vi "CollectPoint.vi"(8 "error in (no error)":errorcluster, 11 "Snake in":refnum<class "SnakeGame.lvclass">) -> (0 "error out":errorcluster, 3 "Snake out":refnum<class "SnakeGame.lvclass">)   [LabVIEW 2019, in "RT_Game.lvlib" / "SnakeGame.lvclass"]
uses:
  SnakeGame.lvclass
  SnakeGame.lvclass/SnakeGame.ctl
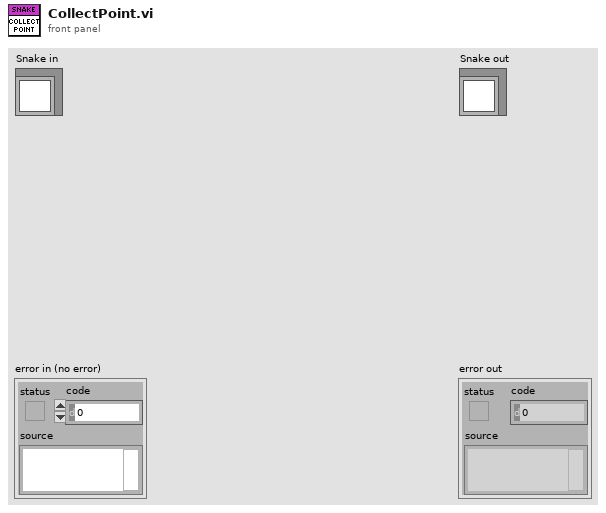
[diagram p1: front panel]
types:
  T1 = typedef "RT_Game.lvlib/Game.lvclass/Coordinate.ctl" = cluster{"x":dbl, "y":dbl}
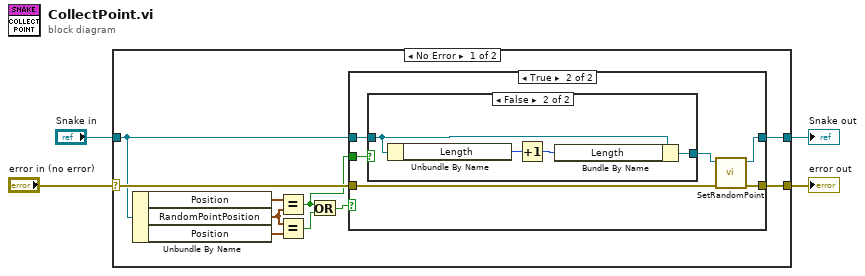
[diagram p0: block diagram]
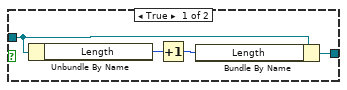
[diagram p3: hidden frame]
diagram:
  n1 = case shown="No Error" "error in (no error)" {
    selector: "error in (no error)" -> [w14 w32]
    tunnel: [w12 w32] -> w3
    tunnel: [w11 w31] -> w1
    tunnel: "Snake in" -> [w10 w31]
    frame No Error {
      n2 = Unbundle By Name(w10) -> ("Position"=w13:T1, "RandomPointPosition"=w9:T1, "Position"=w8:T1)
      n3 = Equal?(x=w13, y=w9) -> (x = y?=w5:bool)
      n4 = Equal?(x=w9, y=w8) -> (x = y?=w6:bool)
      n5 = Or(x=w5, y=w6) -> (x .or. y?=w7:bool)
      n6 = case shown="True" w7 {
        tunnel: w14 -> [w15 w22]
        tunnel: [w15 w21] -> w12
        tunnel: [w16 w20] -> w11
        tunnel: w10 -> [w16 w18]
        tunnel: w5 -> [_ w17]
        frame False {
        }
        frame True {
          n7 = case shown="False" w17 {
            tunnel: [w26 w30] -> w19
            tunnel: w18 -> [w25 w29]
            frame True {
              n8 = Unbundle By Name(w25) -> ("Length"=w24:i16)
              n9 = Increment(x=w24) -> (x+1=w23:i16)
              n10 = Bundle By Name(cluster=w25, "Length"=w23) -> (w26:refnum<class "SnakeGame.lvclass">)
            }
            frame False {
              n11 = Unbundle By Name(w29) -> ("Length"=w28:i16)
              n12 = Increment(x=w28) -> (x+1=w27:i16)
              n13 = Bundle By Name(cluster=w29, "Length"=w27) -> (w30:refnum<class "SnakeGame.lvclass">)
            }
          }
          n14 = call "SetRandomPoint.vi"("error in (no error)"=w22, "Snake in"=w19) -> ("error out"=w21:errorcluster, "Snake out"=w20:refnum<class "SnakeGame.lvclass">)  [unwired: 8 in]
        }
      }
    }
    frame Error {
    }
  }
  "error out" <- w3
  "Snake out" <- w1
